vi "Screenshot.vi"(8 "error in (no error)":errorcluster, 11 "RGetSourceScreenshot in":refnum<class "RGetSourceScreenshot.lvclass">) -> (0 "error out":errorcluster, 2 "Screenshot":picture, 3 "RGetSourceScreenshot out":refnum<class "RGetSourceScreenshot.lvclass">)   [LabVIEW 2022 SP3, in "obs-websocket-lv.lvlib" / "RGetSourceScreenshot.lvclass"]
uses:
  RGetSourceScreenshot.lvclass
  RGetSourceScreenshot.lvclass/RGetSourceScreenshot.ctl
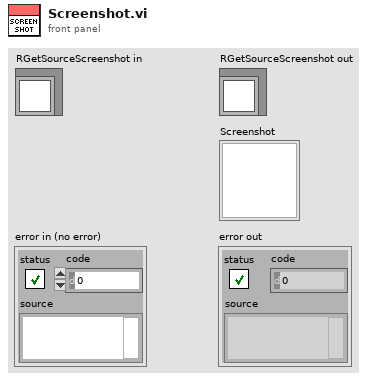
[diagram p1: front panel]
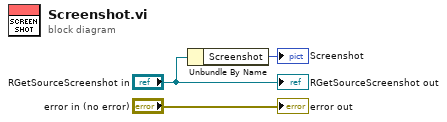
[diagram p0: block diagram]
diagram:
  n1 = Unbundle By Name("RGetSourceScreenshot in") -> ("Screenshot"=→"Screenshot":picture)
  "error out" <- "error in (no error)"
  "RGetSourceScreenshot out" <- "RGetSourceScreenshot in"
